vi "Instrument Type ID.vi"() -> (1 "instrument type id":string="niFGen")   [LabVIEW 2020, in "NI Session Management niFGEN.lvlib"]
uses:
  NI Session Management niFGEN.lvlib
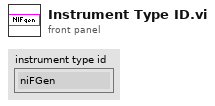
[diagram p1: front panel]
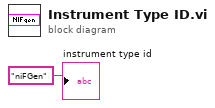
[diagram p0: block diagram]
diagram:
  "instrument type id" <- "niFGen" ("instrument type id")
